vi "上传数据转换.vi"(9 "下位机消息":T1(array[cluster]), 11 "多列列表框":refnum<vi>) -> ()   [LabVIEW 2016]
panel:
  out "项名":string[][](array[string])
  out "数组":u8[](array[numeric])
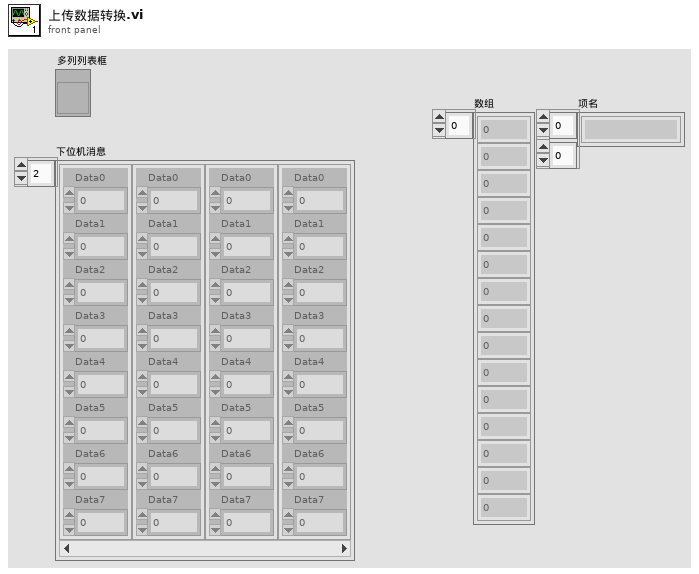
[diagram p1: front panel]
types:
  T1 = cluster{"Data0":u8, "Data1":u8, "Data2":u8, "Data3":u8, "Data4":u8, "Data5":u8, "Data6":u8, "Data7":u8}[]
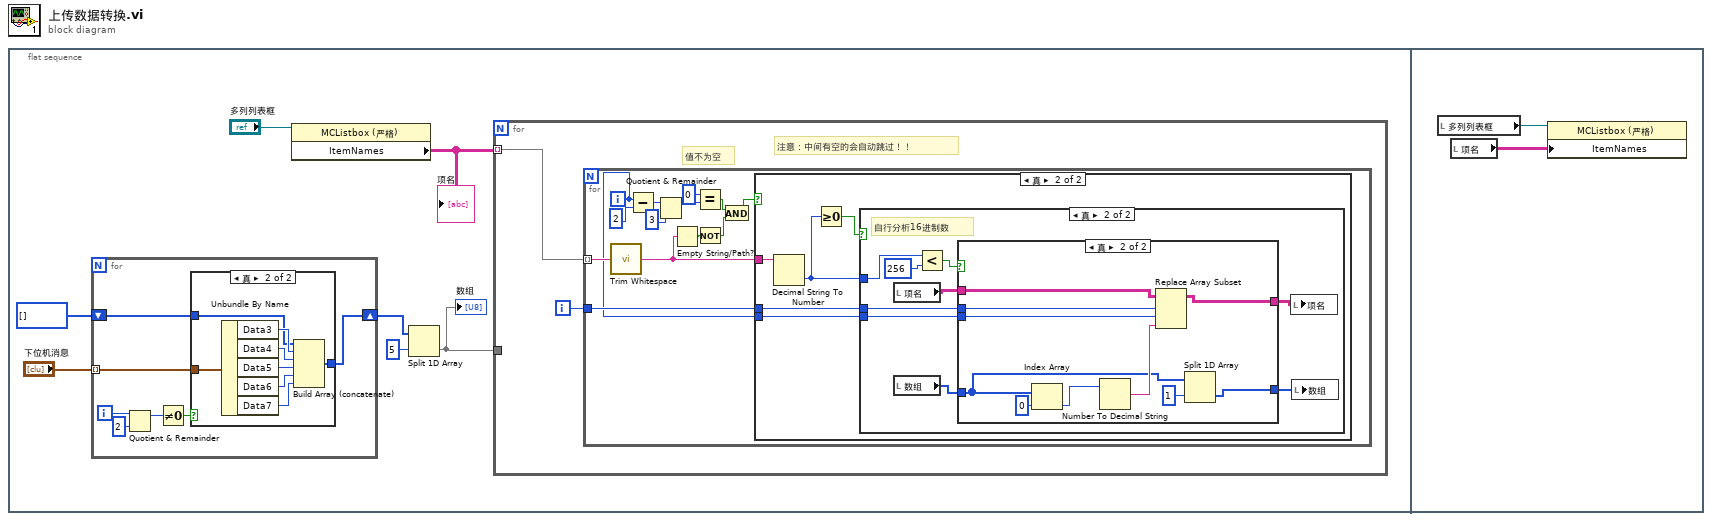
[diagram p0: block diagram]
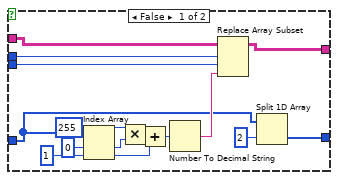
[diagram p4: hidden frame]
diagram:
  n1 = flat-sequence {
    frame #0 {
      n2 = for {
        tunnel: "下位机消息" -> [w64] mode=indexing
        shift-right: [w63] -> w3
        shift-left: u8[] [] -> [w62]
        i -> [w68]
        n3 = Quotient & Remainder(x=w68, y=2) -> (x-y*floor(x/y)=w65:i32)  [unwired: 1 out]
        n4 = Not Equal To 0?(x=w65) -> (x != 0?=w66:bool)
        n5 = case shown="真" w66 {
          tunnel: w64 -> [_ w77]
          tunnel: [w69 w71] -> w63
          tunnel: w62 -> [w69 w70]
          frame False {
          }
          frame True {
            n6 = Unbundle By Name(w77) -> ("Data3"=w76:u8, "Data4"=w75:u8, "Data5"=w74:u8, "Data6"=w73:u8, "Data7"=w72:u8)
            n7 = Build Array (concatenate)(w70, w76, w75, w74, w73, w72) -> (w71:u8[])
          }
        }
      }
      n8 = property class="MCListbox (严格)"(reference="多列列表框") -> ("ItemNames"=w4:string[][])  [unwired: 1 in, 2 out]
      "项名" <- w4
      n9 = Split 1D Array(array=w3, index=5 ("索引")) -> (second subarray=w2:u8[])  [unwired: 1 out]
      "数组" <- w2
      n10 = for {
        tunnel: w4 -> [w9] mode=indexing
        tunnel: w2 -> [_]
        i -> [w8]
        # "注意：中间有空的会自动跳过！！"
        # "值不为空"
        n11 = for {
          tunnel: w9 -> [w17] mode=indexing
          tunnel: w8 -> [w11]
          i -> [w10]
          n12 = call <vilib>:"Trim Whitespace.vi"("string"=w17) -> ("trimmed string"=w16:string)  [unwired: 1 in]
          n13 = Subtract(x=w10, y=2) -> (x-y=w21:i32)
          n14 = Quotient & Remainder(x=w21, y=3) -> (x-y*floor(x/y)=w19:i32)  [unwired: 1 out]
          n15 = Empty String/Path?(string/path=w16) -> (empty?=w15:bool)
          n16 = Equal?(x=0, y=w19) -> (x = y?=w13:bool)
          n17 = Not(x=w15) -> (.not. x?=w14:bool)
          n18 = And(x=w13, y=w14) -> (x .and. y?=w12:bool)
          n19 = case shown="真" w12 {
            tunnel: w16 -> [_ w27]
            tunnel: w11 -> [_ w24]
            tunnel: w10 -> [_ w23]
            frame False {
            }
            frame True {
              n20 = Decimal String To Number(string=w27) -> (number=w25:i32)  [unwired: 2 in, 1 out]
              n21 = Greater Or Equal To 0?(x=w25) -> (x >= 0?=w26:bool)
              n22 = case shown="真" w26 {
                tunnel: w25 -> [_ w36]
                tunnel: w24 -> [_ w33]
                tunnel: w23 -> [_ w32]
                frame False {
                }
                frame True {
                  # "自行分析16进制数"
                  n23 = local read "项名"() -> (w31:string[][])
                  n24 = local read "数组"() -> (w29:u8[])
                  n25 = Less?(x=w36, y=256) -> (x < y?=w34:bool)
                  n26 = case shown="真" w34 {
                    tunnel: w33 -> [w51 w61]
                    tunnel: w32 -> [w50 w60]
                    tunnel: w31 -> [w49 w55]
                    tunnel: [w37 w54] -> w30
                    tunnel: w29 -> [w45 w53]
                    tunnel: [w43 w52] -> w28
                    frame False {
                      n27 = Index Array(array=w45, index #1=0 ("索引"), index #2=1 ("索引")) -> (element #1=w42:u8, element #2=w39:u8)
                      n28 = Multiply(x=u8 255, y=w42) -> (x*y=w40:u8)
                      n29 = Add(x=w40, y=w39) -> (x+y=w38:u8)
                      n30 = Number To Decimal String(number=w38) -> (decimal integer string=w48:string)  [unwired: 1 in]
                      n31 = Replace Array Subset(array=w49, new element=w48, index (row)=w51, index (col)=w50) -> (w37:string[][])
                      n32 = Split 1D Array(array=w45, index=2 ("索引")) -> (second subarray=w43:u8[])  [unwired: 1 out]
                    }
                    frame True {
                      n33 = Index Array(array=w53, index=0 ("索引")) -> (element=w57:u8)
                      n34 = Number To Decimal String(number=w57) -> (decimal integer string=w59:string)  [unwired: 1 in]
                      n35 = Replace Array Subset(array=w55, new element=w59, index (row)=w61, index (col)=w60) -> (w54:string[][])
                      n36 = Split 1D Array(array=w53, index=1 ("索引")) -> (second subarray=w52:u8[])  [unwired: 1 out]
                    }
                  }
                  n37 = local write "项名"(w30) -> ()
                  n38 = local write "数组"(w28) -> ()
                }
              }
            }
          }
        }
      }
    }
    frame #1 {
      n39 = local read "多列列表框"() -> (w79:refnum<vi>)
      n40 = local read "项名"() -> (w78:string[][])
      n41 = property class="MCListbox (严格)"(reference=w79, "ItemNames"=w78) -> ()  [unwired: 1 in, 2 out]
    }
  }
